vi "EjemploArregloWVS.vi"() -> ()   [LabVIEW 2020]
panel:
  out "min value":dbl
  out "max value":dbl
  out "Waveform Graph":waveform(dbl)(graph)
  in  "stop":bool
  in  "Serial":dbl(slide) scale=0.0..10.0
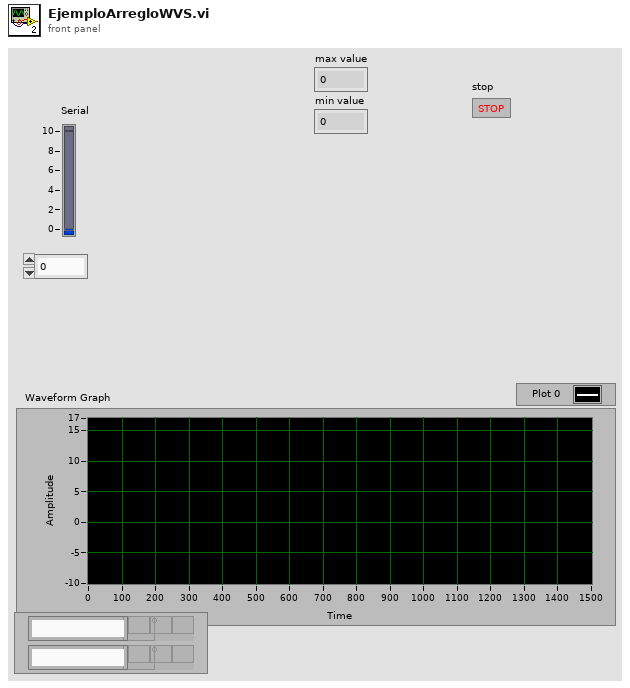
[diagram p1: front panel]
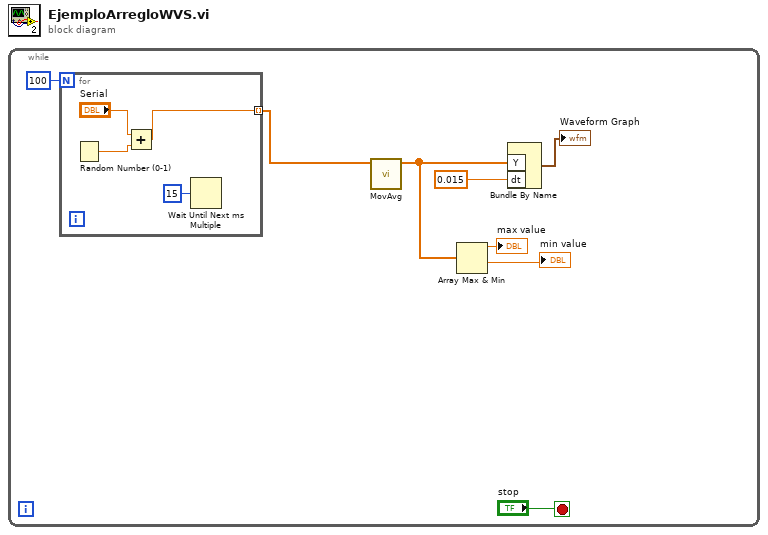
[diagram p0: block diagram]
diagram:
  n1 = while {
    stop <- "stop" stop-if-true
    n2 = for {
      N: 100 -> [_]
      tunnel: [w11] -> w4 mode=indexing
      n3 = Random Number (0-1)() -> (number: 0 to 1=w9:dbl)
      n4 = Add(x="Serial", y=w9) -> (x+y=w11:dbl)
      n5 = Wait Until Next ms Multiple(millisecond multiple=u32 15) -> ()  [unwired: 1 out]
    }
    n6 = call "MovAvg.vi"("Array in"=w4) -> ("Array out"=w1:dbl[])  [unwired: 10 in]
    n7 = Array Max & Min(array=w1) -> (max value=→"max value":dbl, min value=→"min value":dbl)  [unwired: 2 out]
    n8 = Bundle By Name("Y"=w1, "dt"=0.015) -> (→"Waveform Graph":waveform(dbl))  [unwired: 1 in]
  }
